vi "PH_BL-Master.get Status of Status Service Subscriber.vi"(0 "i ref in":refnum<vi>, 2 "Wanted Status Subscriber Information":T1, 5 "error in (no error)":errorcluster) -> (14 "i ref out":refnum<vi>, 15 "off/false/out?":bool, 16 "on/true/in?":bool, 17 "Status":T3 items=["no info", "off/false/out", "on/true/in", "Failure", "Alarm", "Status 1", "Status 2", "Status 3"], 18 "off/false/out or on/true/in?":bool, 19 "error out":errorcluster)   [LabVIEW 2014, in "PH_BL-Master.lvlib"]
doc: "This VI gets the status of the selected Subscriber."
uses:
  PH_BL-Master.lvlib
  PH_StatusHandler/PH_StatusHandler.Status.ctl
  PH_BL-Master.Status Subscriber Information.ctl
  PH_BL-Master.Attribute Set.ctl
  PH_StatusHandler/PH_StatusHandler.lvlib
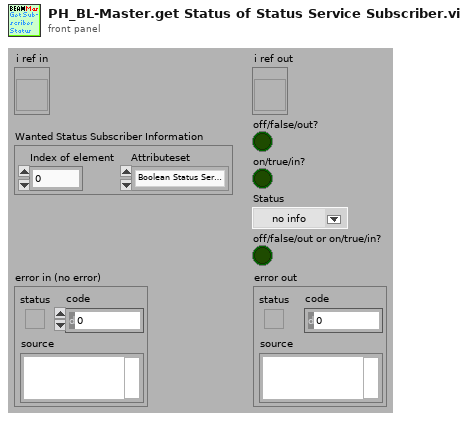
[diagram p1: front panel]
types:
  T1 = typedef "PH_BL-Master.lvlib/PH_BL-Master.Status Subscriber Information.ctl" = cluster{"Index of element":i32, "Attributeset":T2}
  T2 = typedef "PH_BL-Master.lvlib/PH_BL-Master.Attribute Set.ctl" = enum16{"Boolean Status Service Subscriber", "Picture Status Service Subscriber"}
  T3 = typedef "PH_StatusHandler.lvlib/PH_StatusHandler.Status.ctl" = i16
  T4 = typedef "PH_BL-Master.lvlib/PH_BL-Master.i attribute.ctl" = cluster{"Remote controlled":bool, "Boolean Condition Service Subscriber":refnum<vi>[], "Picture Condition Service Subscriber":refnum<vi>[], "R2S":cluster{"GUI Ref":refnum<vi>, "State":bool}, "Vacua":cluster{"GUI Ref":refnum<vi>, "Limit":dbl, "Curr Value":dbl, "in range":bool}[], "O2 Inspection":cluster{"GUI Ref":refnum<vi>, "Concentration":dbl, "State":T3}[], "Boolean Status Service Subscriber":cluster{"GUI Ref":refnum<vi>, "Status":T3, "no Link?":bool, "Status Subscriber Class":T5}[], "Picture Status Service Subscriber":cluster{"GUI Ref":refnum<vi>, "Status":T3, "no Link?":bool, "Status Subscriber Class":T5}[], "6P 4Q Service Subscriber":cluster{"GUI Ref":refnum<vi>, "Selector":T6, "no Link?":bool}[], "Index of latest 6P 4Q changing Instance":i32, "Index of latest Picture Status changing Instance":i32, "Index of latest Boolean Status changing Instance":i32, "Vision ID on same Node":string, "Start Phase over?":bool, "GUI Ref Delete":refnum<vi>}
  T5 = typedef "PH_BL-Master.lvlib/PH_BL-Master.Status Subscriber Class.ctl" = enum16{"unknown", "Switch", "BB", "6P Switch", "Switch GUI", "Switch and 6P State", "Force Sensor"}
  T6 = typedef "PH_4_Pos_Selector.lvlib/PH_4_Pos_Selector.Position Selector.ctl" = u16
  T7 = cluster{"GUI Ref":refnum<vi>, "Status":T3, "no Link?":bool, "Status Subscriber Class":T5}[]
  T8 = cluster{"GUI Ref":refnum<vi>, "Status":T3, "no Link?":bool, "Status Subscriber Class":T5}
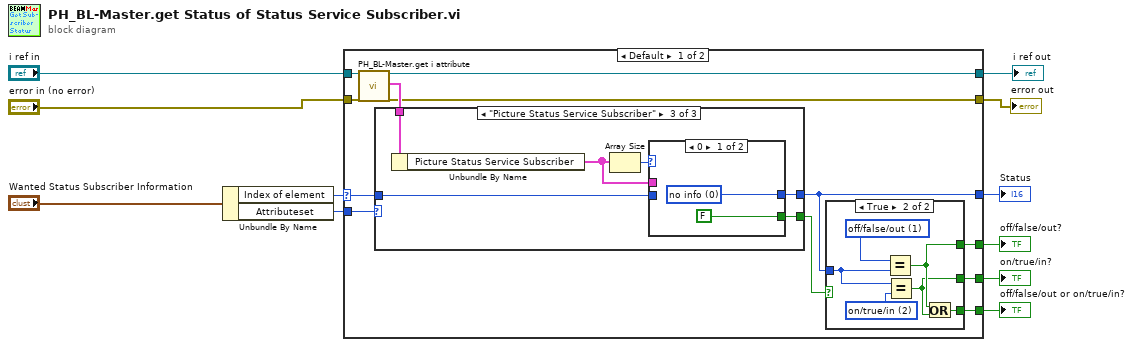
[diagram p0: block diagram]
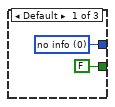
[diagram p2: hidden frame]
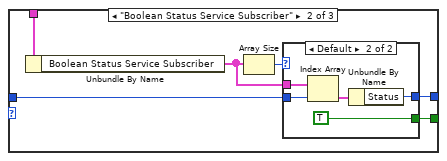
[diagram p3: hidden frame]
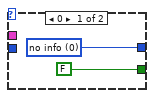
[diagram p4: hidden frame]
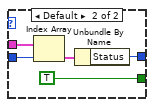
[diagram p5: hidden frame]
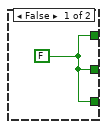
[diagram p6: hidden frame]
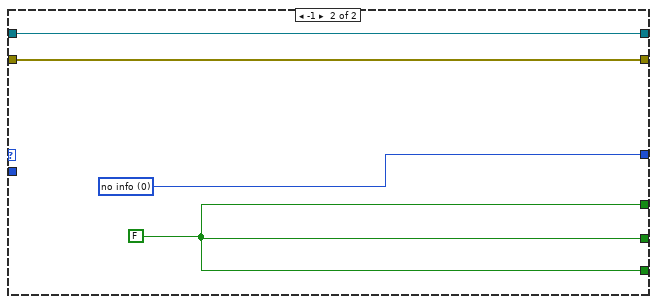
[diagram p7: hidden frame]
diagram:
  n1 = Unbundle By Name("Wanted Status Subscriber Information") -> ("Index of element"=w2:i32, "Attributeset"=w1:T2)
  n2 = case shown="Default" w2 {
    selector: w2 -> [w16 _]
    tunnel: "error in (no error)" -> [w22 w61]
    tunnel: "i ref in" -> [w21 w62]
    tunnel: [w20 w62] -> w4
    tunnel: [w13 w60] -> w6
    tunnel: [w15 w61] -> w5
    tunnel: [w19 w59] -> w7
    tunnel: [w18 w59] -> w8
    tunnel: [w17 w59] -> w9
    tunnel: w1 -> [w14 _]
    frame Default {
      n3 = call "PH_BL-Master.get i attribute.vi"("i ref in"=w21, "error in (no error)"=w22) -> ("i ref out"=w20:refnum<vi>, "i attribute"=w23:T4, "error out"=w15:errorcluster)  [unwired: 15 in]
      n4 = case shown="\"Picture Status Service Subscriber\"" w14 {
        tunnel: w23 -> [_ w31 w44]
        tunnel: w16 -> [_ w28 w41]
        tunnel: [w25 w27 w40] -> w13
        tunnel: [FALSE w26 w39] -> w12
        frame Default {
          w25 = T3 0 items=["no info", "off/false/out", "on/true/in", "Failure", "Alarm", "Status 1", "Status 2", "Status 3"] ("Status")
        }
        frame "Boolean Status Service Subscriber" {
          n5 = Unbundle By Name(w31) -> ("Boolean Status Service Subscriber"=w29:T7)
          n6 = Array Size(array=w29) -> (size(s)=w30:i32)
          n7 = case shown="Default" w30 {
            tunnel: w29 -> [_ w38]
            tunnel: w28 -> [_ w35]
            tunnel: [w33 w36] -> w27
            tunnel: [FALSE TRUE] -> w26
            frame 0 {
              w33 = T3 0 items=["no info", "off/false/out", "on/true/in", "Failure", "Alarm", "Status 1", "Status 2", "Status 3"] ("State")
            }
            frame Default {
              n8 = Index Array(array=w38, index=w35) -> (element=w37:T8)
              n9 = Unbundle By Name(w37) -> ("Status"=w36:T3)
            }
          }
        }
        frame "Picture Status Service Subscriber" {
          n10 = Unbundle By Name(w44) -> ("Picture Status Service Subscriber"=w42:T7)
          n11 = Array Size(array=w42) -> (size(s)=w43:i32)
          n12 = case shown="0" w43 {
            tunnel: w42 -> [_ w51]
            tunnel: w41 -> [_ w48]
            tunnel: [w46 w49] -> w40
            tunnel: [FALSE TRUE] -> w39
            frame 0 {
              w46 = T3 0 items=["no info", "off/false/out", "on/true/in", "Failure", "Alarm", "Status 1", "Status 2", "Status 3"] ("State")
            }
            frame Default {
              n13 = Index Array(array=w51, index=w48) -> (element=w50:T8)
              n14 = Unbundle By Name(w50) -> ("Status"=w49:T3)
            }
          }
        }
      }
      n15 = case shown="True" w12 {
        tunnel: [w52 w57] -> w19
        tunnel: [w52 w56] -> w18
        tunnel: [w52 w55] -> w17
        tunnel: w13 -> [_ w53]
        frame False {
          w52 = FALSE
        }
        frame True {
          w58 = T3 2 items=["no info", "off/false/out", "on/true/in", "Failure", "Alarm", "Status 1", "Status 2", "Status 3"] ("y")
          w54 = T3 1 items=["no info", "off/false/out", "on/true/in", "Failure", "Alarm", "Status 1", "Status 2", "Status 3"] ("y")
          n16 = Equal?(x=w54, y=w53) -> (x = y?=w57:bool)
          n17 = Equal?(x=w53, y=w58) -> (x = y?=w56:bool)
          n18 = Or(x=w57, y=w56) -> (x .or. y?=w55:bool)
        }
      }
    }
    frame -1 {
      w59 = FALSE
      w60 = T3 0 items=["no info", "off/false/out", "on/true/in", "Failure", "Alarm", "Status 1", "Status 2", "Status 3"] ("State")
    }
  }
  "i ref out" <- w4
  "error out" <- w5
  "Status" <- w6
  "off/false/out?" <- w7
  "on/true/in?" <- w8
  "off/false/out or on/true/in?" <- w9
